vi "Test-Ignore.vi"() -> ()   [LabVIEW 2019]
panel:
  in  "stop":bool
  out "Tick Count(uSec)":u32
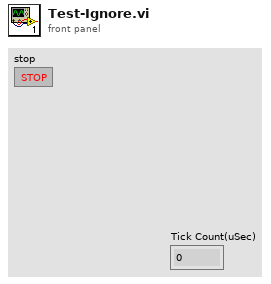
[diagram p1: front panel]
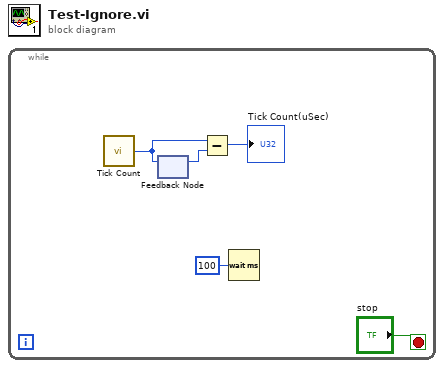
[diagram p0: block diagram]
diagram:
  n1 = while {
    stop <- "stop" stop-if-true
    n2 = call "Tick Count"() -> ("Tick Count(mSec)"=w3:u32)
    n3 = feedback-in #1(w3) -> ()
    n4 = feedback #1() -> (w5:u32)  [unwired: 1 in]
    n5 = Subtract(x=w3, y=w5) -> (x-y=→"Tick Count(uSec)":u32)
    n6 = Wait (ms)(milliseconds to wait=u32 100) -> ()  [unwired: 1 out]
  }
